vi "Connect to Error Handles.vi"(8 "error in":errorcluster, 9 "Timeout (ms)":u16, 11 "Async in":refnum<class "VS Plugin Inline Async API.lvclass">=refnum) -> (0 "error out":errorcluster, 3 "Async out":refnum<class "VS Plugin Inline Async API.lvclass">)   [LabVIEW 2023, in "VS Plugin Inline Async API.lvlib" / "VS Plugin Inline Async API.lvclass"]
uses:
  VS Plugin Inline Async API.lvclass
  VS Plugin Inline Async API.lvclass/VS Plugin Inline Async API.ctl
  VS Plugin Inline Async API.lvlib
  <vilib>/ErrorRing/Error Ring.xnode
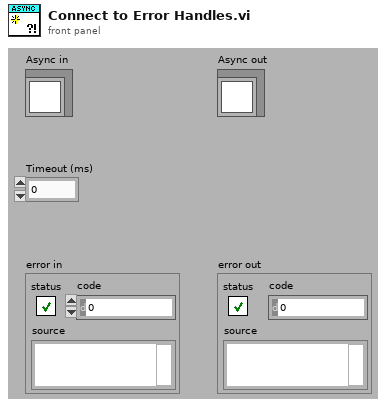
[diagram p1: front panel]
types:
  T1 = cluster{"read mode":enum16{"polling", "blocking"}, "write mode":enum16{"polling", "blocking"}}
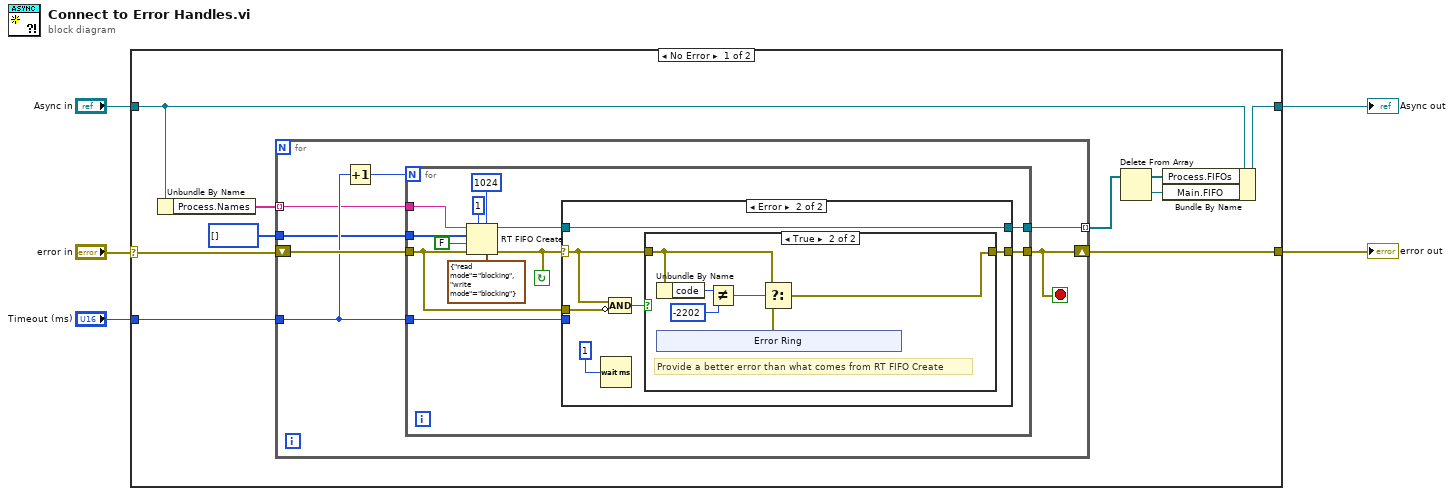
[diagram p0: block diagram]
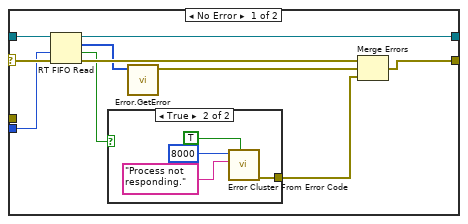
[diagram p2: hidden frame]
diagram:
  n1 = case shown="No Error" "error in" {
    selector: "error in" -> [w14 w67]
    tunnel: [w10 w67] -> w5
    tunnel: "Timeout (ms)" -> [w15 _]
    tunnel: "Async in" -> [w12 w66]
    tunnel: [w13 w66] -> w1
    frame No Error {
      n2 = Unbundle By Name(w12) -> ("Process.Names"=w11:string[])
      n3 = for {
        shift-right: [w17] -> w10
        shift-left: w14 -> [w22]
        tunnel: [w21] -> w9 mode=indexing
        tunnel: w15 -> [w19]
        tunnel: w11 -> [w18] mode=indexing
        tunnel: u8[] [] -> [w16]
        stop <- w17 stop-if-true
        n4 = Increment(x=w19) -> (x+1=w20:u16)
        n5 = for {
          N: w20 -> [_]
          tunnel: [w33] -> w21
          tunnel: w19 -> [w31]
          tunnel: w22 -> [w23]
          tunnel: [w30] -> w17
          tunnel: w18 -> [w28]
          tunnel: w16 -> [w25]
          stop <- w29 continue-if-true
          n6 = RT FIFO Create(0:w28, 1:w25, 2:FALSE ("create if not found? (T)"), 3:w23, 4:u32 1 ("size (10)"), 6:u32 1024 ("elements in array (1)"), 7:T1 {"read mode"=enum."blocking", "write mode"=enum."blocking"} ("r/w modes (polling,polling)")) -> (8:w32:refnum<k33>, 11:w29:errorcluster)  [unwired: 1 in, 1 out]
          n7 = case shown="Error" w29 {
            selector: w29 -> [w42 w50]
            tunnel: [w39 w49] -> w30
            tunnel: [w43 w54] -> w33
            tunnel: w32 -> [w44 w54]
            tunnel: w31 -> [w41 _]
            tunnel: w23 -> [_ w52]
            frame No Error {
              n8 = RT FIFO Read(0:w44, 2:w41, 3:w42) -> (8:w43:refnum<k33>, 9:w35:u8[], 10:w37:bool, 11:w40:errorcluster)  [unwired: 1 in, 1 out]
              n9 = case shown="True" w37 {
                tunnel: [_ w48] -> w38
                frame False {
                }
                frame True {
                  n10 = call <vilib>:"Error Cluster From Error Code.vi"("show call chain? (False)"=TRUE, "error message (\"\")"="Process not responding." ("source"), "error code (0)"=8000) -> ("error out"=w48:errorcluster)  [unwired: 6 in]
                }
              }
              n11 = call "Error.GetError.vi"("Msg"=w35) -> ("error out"=w36:errorcluster)  [unwired: 10 in]
              n12 = Merge Errors(w40, w36, w38) -> (w39:errorcluster)
            }
            frame Error {
              n13 = Wait (ms)(milliseconds to wait=u32 1) -> ()  [unwired: 1 out]
              n14 = Compound Arithmetic op=AND(w50, invert w52) -> (w51:bool)
              n15 = case shown="True" w51 {
                tunnel: w50 -> [w55 w58]
                tunnel: [w55 w56] -> w49
                frame False {
                  # "No new error from RT FIFO Create"
                }
                frame True {
                  # "Provide a better error than what comes from RT FIFO Create"
                  n16 = Unbundle By Name(w58) -> ("code"=w61:i32)
                  n17 = xnode "Error Ring"() -> ("error out"=w57:errorcluster)
                  n18 = Not Equal?(x=w61, y=-2202) -> (x != y?=w59:bool)
                  n19 = Select(t=w58, s=w59, f=w57) -> (s? t:f=w56:errorcluster)
                }
              }
            }
          }
        }
      }
      n20 = Delete From Array(array=w9) -> (deleted portion=w8:refnum<k33>, array with subset deleted=w7:refnum<k33>[])  [unwired: 2 in]
      n21 = Bundle By Name(cluster=w12, "Process.FIFOs"=w7, "Main.FIFO"=w8) -> (w13:refnum<class "VS Plugin Inline Async API.lvclass">)
    }
    frame Error {
    }
  }
  "error out" <- w5
  "Async out" <- w1
